vi "Calibration-Line3-CalMain.vi"(8 "error in (no error)":errorcluster, 11 "Calibration-RunTest in":refnum<class "Calibration-RunTest.lvclass">) -> (0 "error out":errorcluster, 3 "Calibration-RunTest out":refnum<class "Calibration-RunTest.lvclass">)   [LabVIEW 2013, in "Calibration-RunTest.lvclass"]
uses:
  Calibration-RunTest.lvclass
  Calibration-RunTest.lvclass/Calibration-RunTest.ctl
  Motion Control/Motion-ControlAll.lvclass
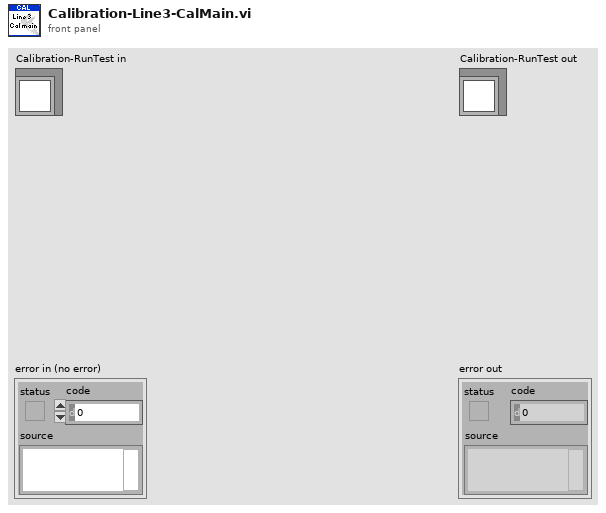
[diagram p1: front panel]
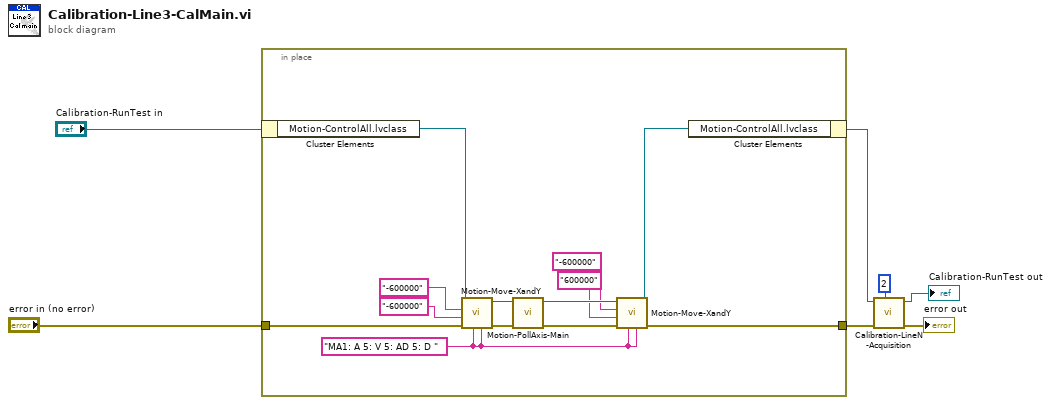
[diagram p0: block diagram]
diagram:
  n1 = in-place {
    in-place-border: "error in (no error)" -> [w11]
    in-place-border: [w8] -> w4
    w9 = "MA1: A 5: V 5: AD 5: D " ("concatenated string")
    n2 = in-place-cluster #1("Calibration-RunTest in") -> ("Motion-ControlAll.lvclass"=w12:refnum<class "Motion-ControlAll.lvclass">)
    n3 = call "Motion-Move-XandY.vi"("Y Drive Acc/Speed/Velocity"=w9, "X Drive Acc/Speed/Velocity"=w9, "error in (no error)"=w11, "X Coordinates"="-600000", "Y Coordinates"="-600000", "Motion-ControlAll in"=w12) -> ("error out"=w14:errorcluster, "Motion-ControlAll out"=w13:refnum<class "Motion-ControlAll.lvclass">)  [unwired: 4 in]
    n4 = call "Motion-PollAxis-Main.vi"("error in (no error)"=w14, "Motion-ControlAll in"=w13) -> ("error out"=w19:errorcluster, "Motion-ControlAll out"=w20:refnum<class "Motion-ControlAll.lvclass">)  [unwired: 8 in]
    n5 = call "Motion-Move-XandY.vi"("Y Drive Acc/Speed/Velocity"=w9, "X Drive Acc/Speed/Velocity"=w9, "error in (no error)"=w19, "X Coordinates"="600000", "Y Coordinates"="-600000", "Motion-ControlAll in"=w20) -> ("error out"=w8:errorcluster, "Motion-ControlAll out"=w10:refnum<class "Motion-ControlAll.lvclass">)  [unwired: 4 in]
    n6 = in-place-cluster #1("Motion-ControlAll.lvclass"=w10) -> (w3:refnum<class "Calibration-RunTest.lvclass">)
  }
  n7 = call "Calibration-LineN-Acquisition.vi"("Cal Line?"=2, "error in (no error)"=w4, "Calibration-RunTest in"=w3) -> ("error out"=→"error out":errorcluster, "Calibration-RunTest out"=→"Calibration-RunTest out":refnum<class "Calibration-RunTest.lvclass">)  [unwired: 7 in]
